vi "Multi-index 2D Array.vi"(1 "Indices":cluster{"Row":i32, "Column":i32}[](array[cluster]), 2 "Array":dbl[][](array[numeric])) -> (0 "Values":dbl[](array[numeric]))   [LabVIEW 2018]
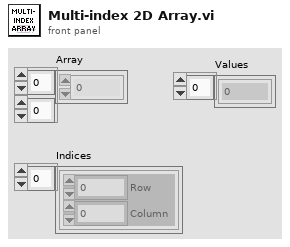
[diagram p1: front panel]
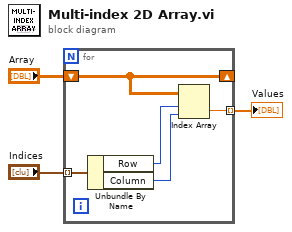
[diagram p0: block diagram]
diagram:
  n1 = for {
    tunnel: "Indices" -> [w8] mode=indexing
    shift-right: [w4] -> _
    shift-left: "Array" -> [w4]
    tunnel: [w5] -> w1 mode=indexing
    n2 = Unbundle By Name(w8) -> ("Row"=w7:i32, "Column"=w6:i32)
    n3 = Index Array(array=w4, index (row)=w7, index (col)=w6) -> (element=w5:dbl)
  }
  "Values" <- w1
